vi "LatchBooleanKeyboardSim.vi"(0 "VI Reference In":refnum<vi>, 1 "Label (VI Title)":string="Default", 11 "error in (no error)":errorcluster) -> (4 "VI Reference Out":refnum<vi>, 15 "error out":errorcluster)   [LabVIEW 2016, in "DronaTest.lvlib"]
uses:
  DronaTest.lvlib
  APIs/Stimulus/ControlValue/ValueSignalLatchBooleanString.vi
  APIs/Assert/AssertControlValue/Equal.vi
  <vilib>/addons/_JKI Toolkits/Caraya/classes/Assert/Assert Not Error.vi
  <vilib>/addons/_JKI Toolkits/Caraya/classes/Test/Test.lvclass
  Drona.lvlib
  <vilib>/addons/_JKI Toolkits/Caraya/classes/Assert/Assert.lvclass
  APIs/Assert/AssertControlValue/AssertControlValue.lvlib
  APIs/Stimulus/ControlValue/ControlValue.lvlib
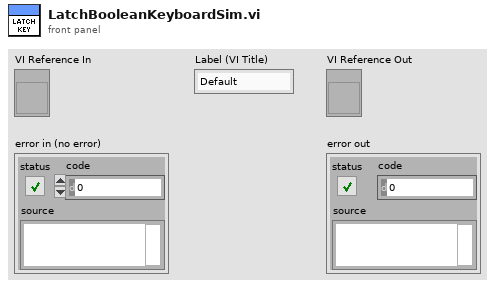
[diagram p1: front panel]
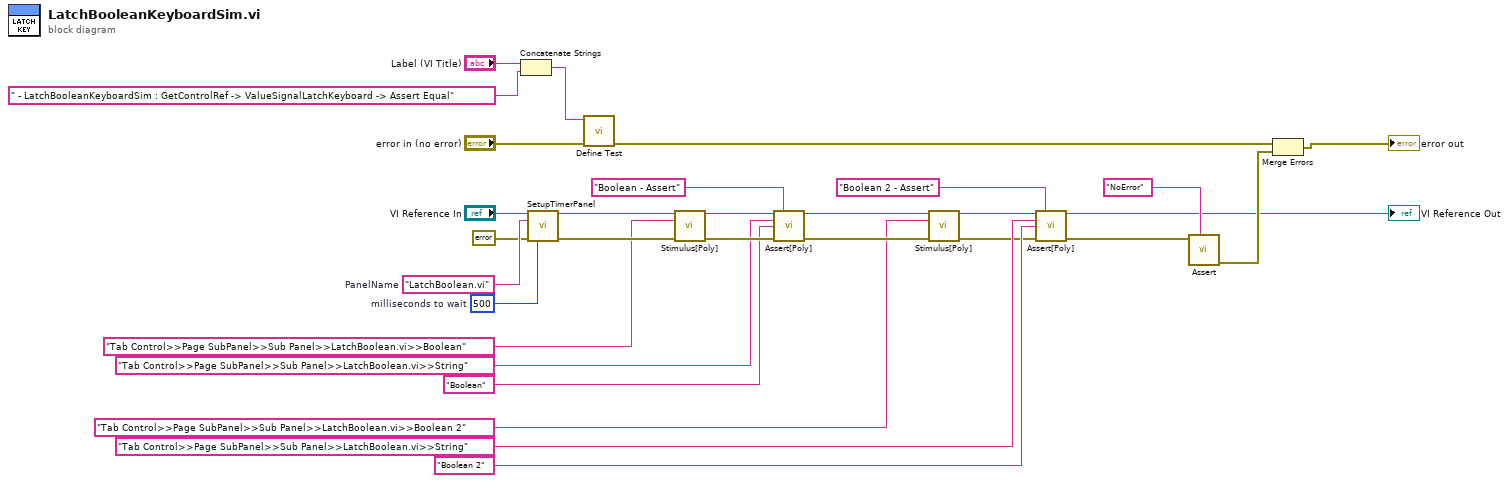
[diagram p0: block diagram]
diagram:
  w3 = u32 500  # milliseconds to wait
  w22 = "LatchBoolean.vi"  # PanelName
  n1 = Concatenate Strings("Label (VI Title)", " - LatchBooleanKeyboardSim : GetControlRef -> ValueSignalLatchKeyboard -> Assert Equal" ("Label (VI Title)")) -> (w24:string)
  n2 = call "SetupTimerPanel.vi"("VI in"="VI Reference In", "Panel Name"=w22, "error in (no error)"=errorcluster {"status"=FALSE, "code"=0, "source"=""} ("error in"), "milliseconds to wait (1000)"=w3) -> ("VI out"=w19:refnum<vi>, "error out"=w5:errorcluster)  [unwired: 10 in]
  n3 = call <vilib>:"Define Test.vi"("error in (no error)"="error in (no error)", "Label (VI Title)"=w24) -> ("error out"=w27:errorcluster)  [unwired: 9 in]
  n4 = call-poly "Stimulus[Poly].vi"("VI Reference In"=w19, "Control Path"="Tab Control>>Page SubPanel>>Sub Panel>>LatchBoolean.vi>>Boolean", "error in"=w5) -> ("VI Reference Out"=w18:refnum<vi>, "error out"=w20:errorcluster)  [unwired: 11 in]
  n5 = call-poly "Assert[Poly].vi"("VI Reference In"=w18, "Test Label"="Boolean - Assert" ("string"), "Control Path"="Tab Control>>Page SubPanel>>Sub Panel>>LatchBoolean.vi>>String", "Control Value"="Boolean" ("Control Path"), "Error In"=w20) -> ("VI Reference Out"=w8:refnum<vi>, "Error Out"=w9:errorcluster)  [unwired: 9 in]
  n6 = call-poly "Stimulus[Poly].vi"("VI Reference In"=w8, "Control Path"="Tab Control>>Page SubPanel>>Sub Panel>>LatchBoolean.vi>>Boolean 2", "error in"=w9) -> ("VI Reference Out"=w11:refnum<vi>, "error out"=w10:errorcluster)  [unwired: 11 in]
  n7 = call-poly "Assert[Poly].vi"("VI Reference In"=w11, "Test Label"="Boolean 2 - Assert" ("string"), "Control Path"="Tab Control>>Page SubPanel>>Sub Panel>>LatchBoolean.vi>>String", "Control Value"="Boolean 2" ("Control Path"), "Error In"=w10) -> ("VI Reference Out"=→"VI Reference Out":refnum<vi>, "Error Out"=w6:errorcluster)  [unwired: 9 in]
  n8 = call-poly <vilib>:"Assert.vi"("Label"="NoError" ("string"), "Not Error?"=w6) -> ("error out"=w30:errorcluster)  [unwired: 9 in]
  n9 = Merge Errors(w27, w30) -> (→"error out":errorcluster)
